vi "ExponentialAve.vi"(6 "Coff":dbl=0.5 format="%#_13g", 9 "PreviousValue":dbl, 10 "InputValue":dbl) -> (2 "Smoothed Value":dbl)   [LabVIEW 2014]
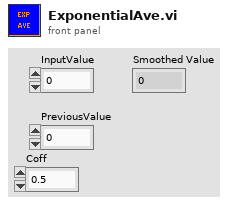
[diagram p1: front panel]
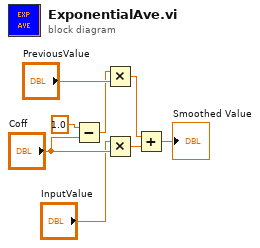
[diagram p0: block diagram]
diagram:
  n1 = Subtract(x=1.0, y="Coff") -> (x-y=w2:dbl)
  n2 = Multiply(x=w2, y="PreviousValue") -> (x*y=w7:dbl)
  n3 = Multiply(x="InputValue", y="Coff") -> (x*y=w6:dbl)
  n4 = Add(x=w7, y=w6) -> (x+y=→"Smoothed Value":dbl)
